vi "TestStop.vi"(8 "error in (no error)":errorcluster) -> (0 "error out":errorcluster)   [LabVIEW 2019]
uses:
  <vilib>/addons/_JKI Toolkits/Caraya/classes/Test/Test.lvclass
  <vilib>/addons/_JKI Toolkits/Caraya/classes/Assert/Assert.lvclass
  <vilib>/addons/_JKI Toolkits/Caraya/classes/Assert/Assert Equal Value_Variant.vi
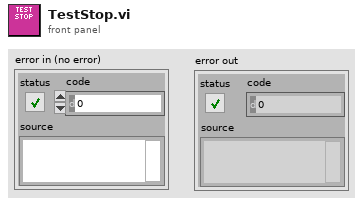
[diagram p1: front panel]
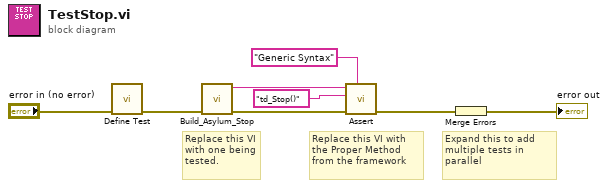
[diagram p0: block diagram]
diagram:
  # "Expand this to add multiple tests in parallel"
  # "Replace this VI with one being tested."
  # "Replace this VI with the Proper Method from the framework"
  n1 = call <vilib>:"Define Test.vi"("error in (no error)"="error in (no error)") -> ("error out"=w4:errorcluster)  [unwired: 10 in]
  n2 = call "Build_Asylum_Stop.vi"("error in (no error)"=w4) -> ("error out"=w3:errorcluster, "Command"=w2:string)  [unwired: 9 in]
  n3 = call-poly <vilib>:"Assert.vi"("Label"="Generic Syntax", "error in (no error)"=w3, "Y"="td_Stop()", "X"=w2) -> ("error out"=w6:errorcluster)  [unwired: 7 in]
  n4 = Merge Errors(w6) -> (→"error out":errorcluster)
